vi "Write Override Data.vi"(8 "error in (no error)":errorcluster, 10 "Override data":T1[](array[typedef]), 11 "Loop Msg in":refnum<class "Loop Msg.lvclass">) -> (0 "error out":errorcluster, 3 "Loop Msg out":refnum<class "Loop Msg.lvclass">)   [LabVIEW 2020, in "Sequencer.lvlib" / "Loop Msg.lvclass"]
doc: "Write Override Data to the class and set the iteration to 0."
uses:
  Loop Msg.lvclass
  Sequence Editor/Controls/Ctl_FlexDataElements.ctl
  Sequence Editor/Controls/Ctl_FlexDataElement.ctl
  Loop Msg.lvclass/Loop Msg.ctl
  Sequencer.lvlib
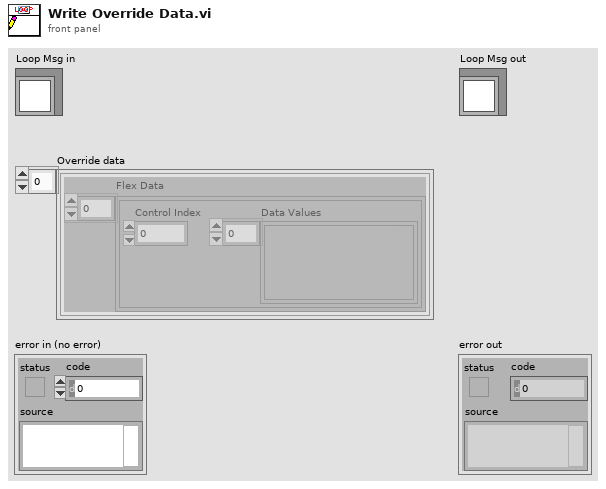
[diagram p1: front panel]
types:
  T1 = typedef "Sequencer.lvlib/Ctl_FlexDataElements.ctl" = cluster{"Flex Data":T2[]}
  T2 = typedef "Sequencer.lvlib/Ctl_FlexDataElement.ctl" = cluster{"Control Index":i32, "Data Values":variant[]}
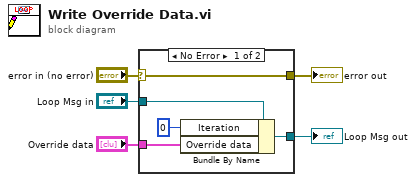
[diagram p0: block diagram]
diagram:
  n1 = case shown="No Error" "error in (no error)" {
    selector: "error in (no error)" -> [w10 w11]
    tunnel: [w10 w11] -> w4
    tunnel: [w8 w12] -> w2
    tunnel: "Loop Msg in" -> [w9 w12]
    tunnel: "Override data" -> [w6 _]
    frame No Error {
      n2 = Bundle By Name(cluster=w9, "Iteration"=0, "Override data"=w6) -> (w8:refnum<class "Loop Msg.lvclass">)
    }
    frame Error {
    }
  }
  "error out" <- w4
  "Loop Msg out" <- w2
